vi "TagRouter.vi"(7 "Name(\"\" to use uuid)":string="UI.Dashboard") -> ()   [LabVIEW 2020, in "CSM-TagRouter.lvlib"]
doc: "------------- lvcsm -------------\n[CSMStates]\nItem 0 = \"Idle\"\nItem 1 = \"CSM Documentation\"\nItem 2 = \"VI Reference\"\nItem 3 = \"Error Handler\"\nItem 4 = \"Critical Error\"\nItem 5 = \"Target Timeout Error\"\nItem 6 = \"Target Error\"\nItem 7 = \"Async Response\"\nItem 8 = \"Response\"\nItem 9 = \"Async Message Posted\"\nItem 10 = \"Initialize Core Data\"\nItem 11 = \"Exit\"\nItem 12 = \"Data: Initialize\"\nItem 13 = \"Data: Update Indicators\"\nItem 14 = \"Data: Load Attributes\"\nItem 15 = \"Data: Save Attributes\"\nItem 16 = \"Data: Cleanup\"\nItem 17 = \"Macro: Initialize\"\nItem 18 = \"Macro: Exit\"\nItem 19 = \"API: Start Refreshing\"\nItem 20 = \"API: Stop Refreshing\"\nItem 21 = \"Action: Insert TestStandOI\"\nItem 22 = \"Action: Relocate Boolean Switchs\"\nItem 23 = \"Action: 修改bool状态\"\nItem 24 = \"Action: Sync Bool Value with DB\"\nItem 25 = \"Action: 更新当前测试名称\"\nItem 26 = \"Action: Refresh Waveform\"\nItem 27 = \"Action: Refresh Check\"\nItem 28 = \"Action: Resize Array\"\n\n[CSMStatus]\nItem 0 = \"Error Occurred@Error Handler\"\nItem 1 = \"电磁阀状态修改@Action: 修改bool状态\""
uses:
  CSM-TagRouter.lvlib
  ee6b4457-3910-401d-b6a0-627ba86d4b6e.vi
  9c140fab-bc64-4413-82a8-cd8ed97da630.vi
  82eb00db-d07c-457e-bb6f-b363662c3af2.vi
  cb63b056-b8cb-4b3f-bf45-ca82b840c7fe.vi
  edf08d9e-89a8-4fbb-bbaf-5d87ab7e3973.vi
  <userlib>/_NEVSTOP/Communicable State Machine(CSM)/AdvanceAPI/CSM - Revert Arguments-Safe String.vi
  <userlib>/_NEVSTOP/Communicable State Machine(CSM)/_Shared/Trim Single-line Text.vi
  <userlib>/_NEVSTOP/Communicable State Machine(CSM)/AdvanceAPI/CSM - Make String Arguments Safe.vi
  <userlib>/_NEVSTOP/Communicable State Machine(CSM)/AdvanceAPI/CSM - Break Down Multiple States String.vi
  <userlib>/_NEVSTOP/Communicable State Machine(CSM)/AdvanceAPI/CSM - Compact Multiple States.vi
  <userlib>/_NEVSTOP/TagDB/_Support/DataAccess/data-Write.vi
  <userlib>/_NEVSTOP/TagDB/_Support/Error/_[error50000]Invalid DB REF.vi
  <userlib>/_NEVSTOP/TagDB/_Support/DataAccess/TagDB Ref to DVR.vi
  <userlib>/_NEVSTOP/Communicable State Machine(CSM)/AdvanceAPI/CSM - Keywords.vi
  <userlib>/_NEVSTOP/TagDB/_Support/DataAccess/_NameCacher.vi
  <userlib>/_NEVSTOP/TagDB/_Support/DataAccess/_datatypeChecker.vi
  <vilib>/Utility/Data Type/Get Type Information.vi
  <userlib>/_NEVSTOP/TagDB/_Support/Error/_Build Error Cluster.vi
  <userlib>/_NEVSTOP/Communicable State Machine(CSM)/addons/MassData-Parameter/_support/FGV-MassData(lvlibp).vi
  <userlib>/_NEVSTOP/Communicable State Machine(CSM)/addons/API-String-Arugments-Support/_Support/Data To API String Arguments.vi
  <userlib>/_NEVSTOP/Communicable State Machine(CSM)/Communicable State Machine.lvlib
  <userlib>/_NEVSTOP/TagDB/TagDB.lvlib
  <userlib>/_NEVSTOP/Communicable State Machine(CSM)/addons/API-String-Arugments-Support/API String Arguments Support.lvlib
  <userlib>/_NEVSTOP/Communicable State Machine(CSM)/_Shared/CSM Shared.lvlib
panel:
  out "TagDB":refnum<k1>
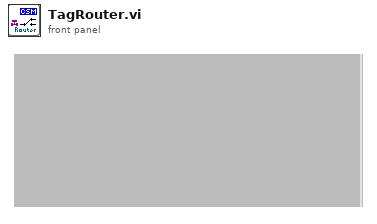
[diagram p1: front panel]
types:
  T1 = enum32{"Invalid", "Standard", "Closed", "Hidden", "Minimized", "Maximized"}
  T2 = enum32{"invalid app kind", "Development System", "Run Time System", "Student Edition", "Embedded LabVIEW", "Evaluation", "Custom"}
  T3 = typedef "Communicable State Machine.lvlib/_CSM_Response Source Message.ctl" = cluster{"‘State":string, "’Arguments":string, "’Error":errorcluster}
  T4 = cluster{"Current VI Reference":refnum<vi>, "Close Panel on Exit?":bool}
  T5 = cluster{"Core":cluster{"Current VI Reference":refnum<vi>, "Close Panel on Exit?":bool}, "Tags":string[], "Size":cluster{"Cols":i16, "Rows":i16}}
  T6 = cluster{"NI_DeviceNumber":string, "NI_ChannelName":string, "NI_LineNames":string, "NI_UnitDescription":string, "NI_ExpXDimension":string}
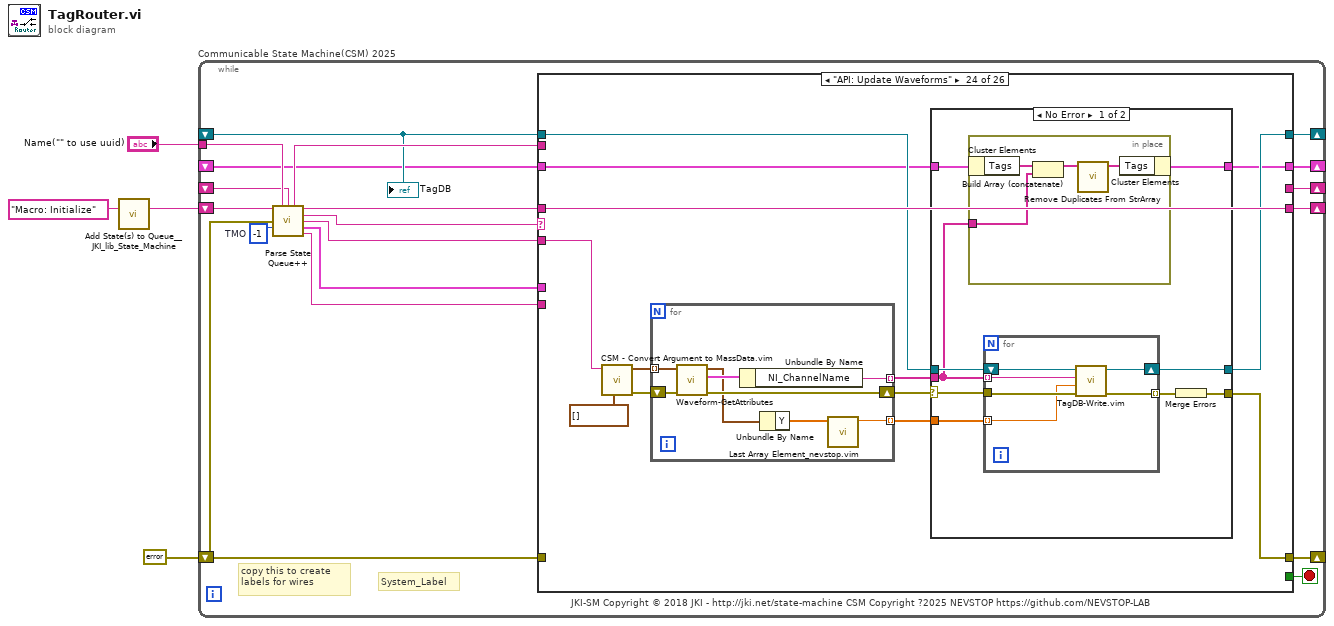
[diagram p0: block diagram]
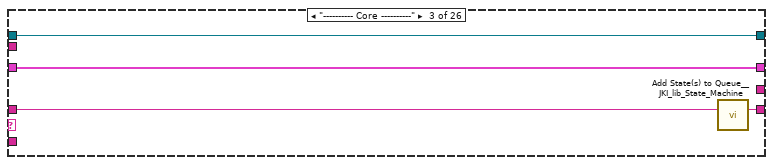
[diagram p4: hidden frame]
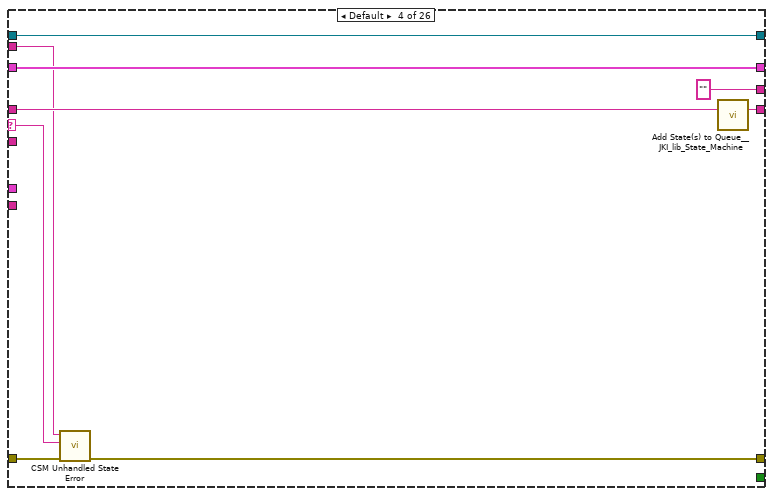
[diagram p5: hidden frame]
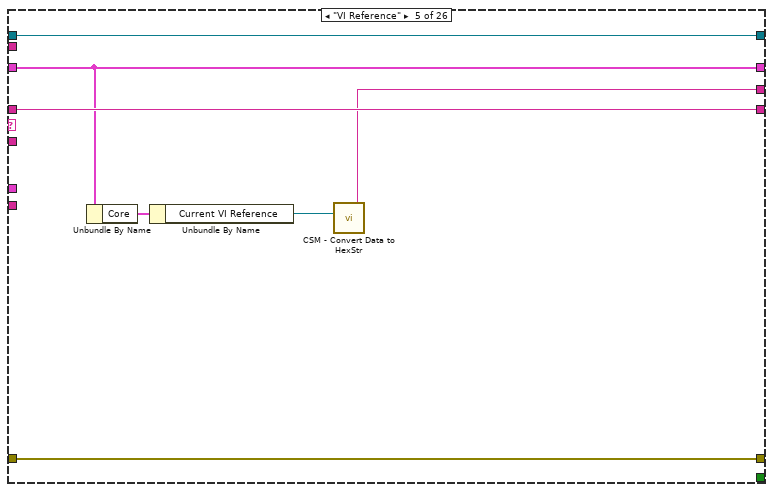
[diagram p6: hidden frame]
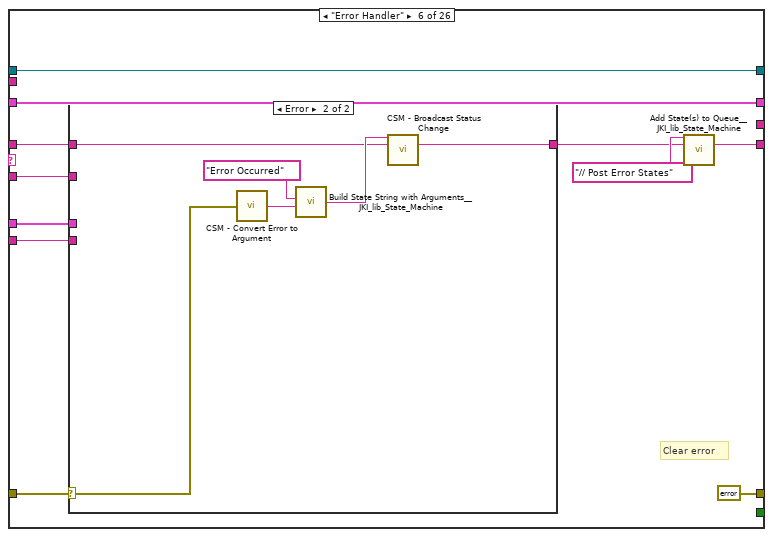
[diagram p7: hidden frame]
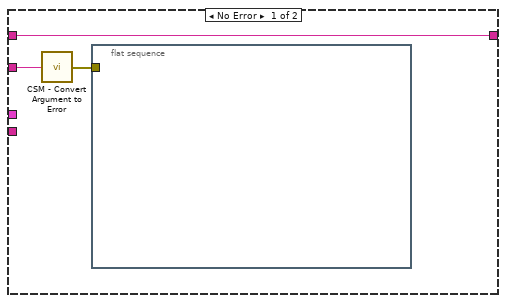
[diagram p8: hidden frame]
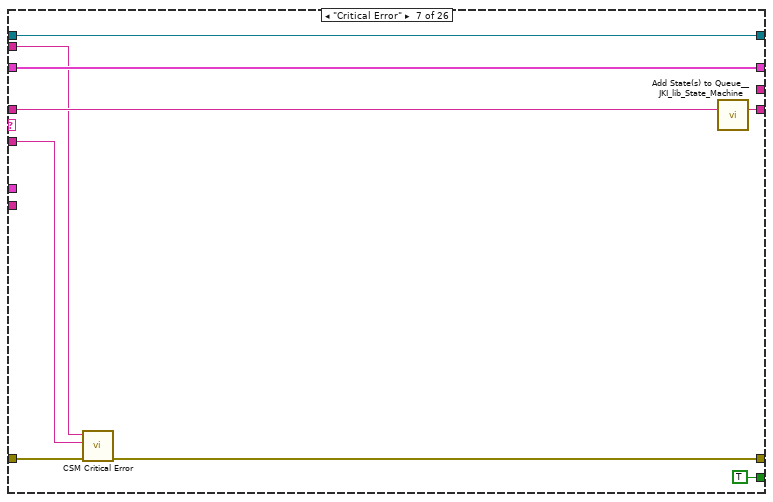
[diagram p9: hidden frame]
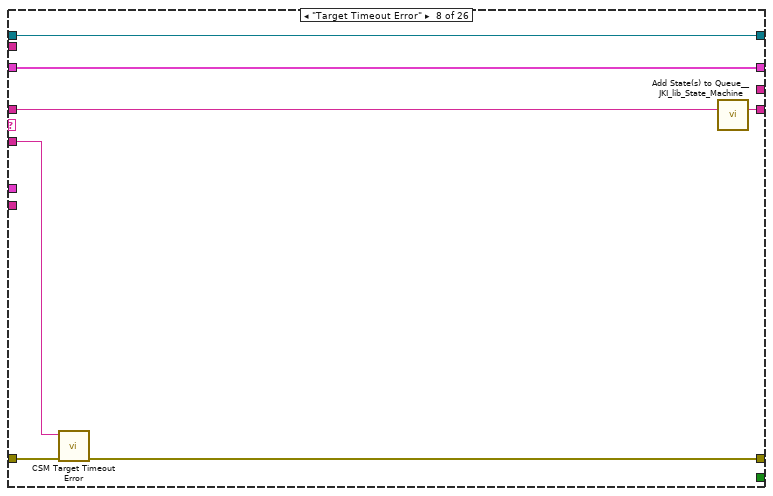
[diagram p10: hidden frame]
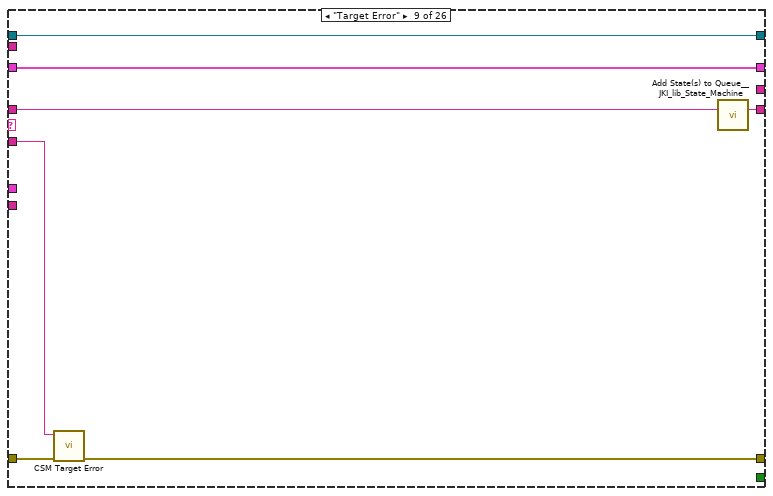
[diagram p11: hidden frame]
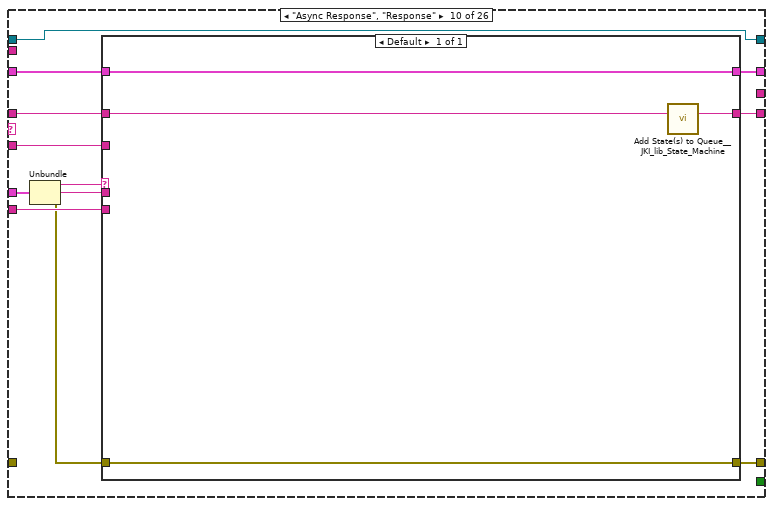
[diagram p12: hidden frame]
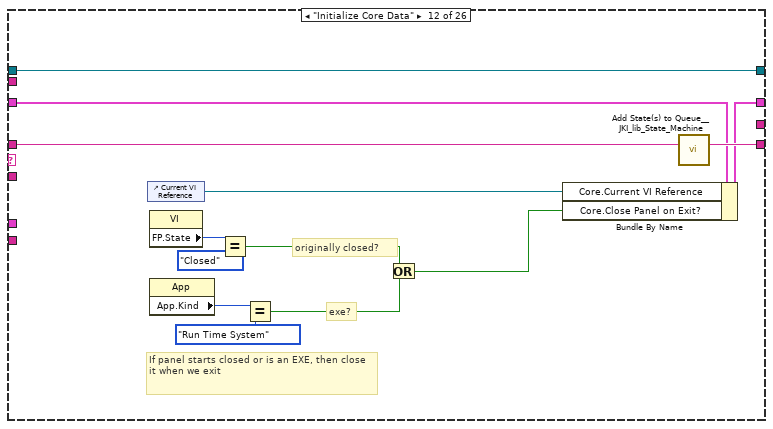
[diagram p14: hidden frame]
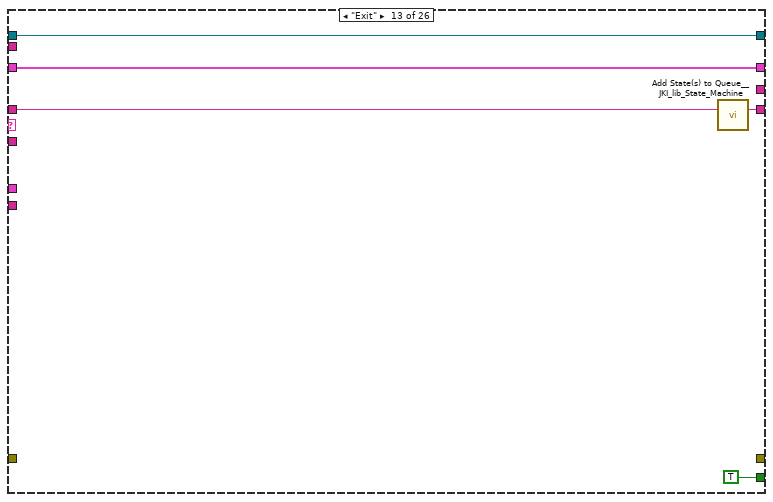
[diagram p15: hidden frame]
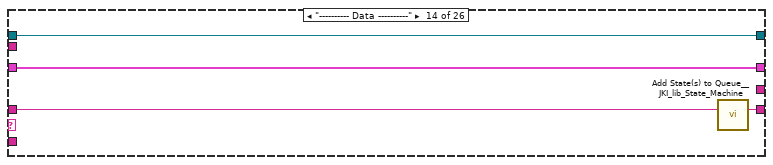
[diagram p16: hidden frame]
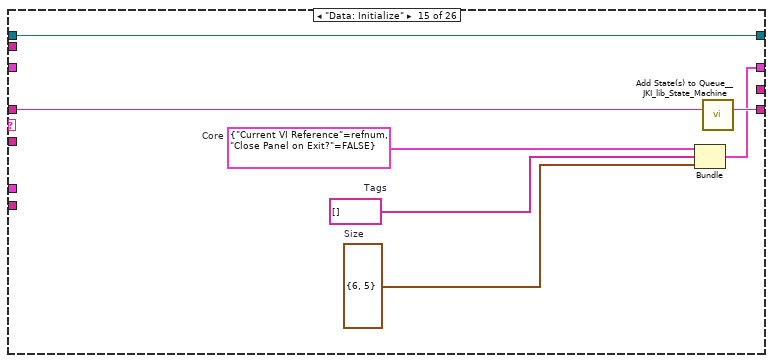
[diagram p17: hidden frame]
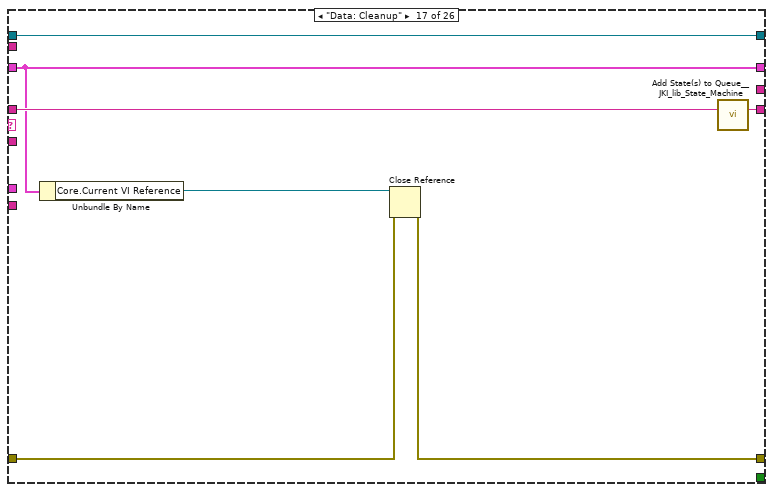
[diagram p19: hidden frame]
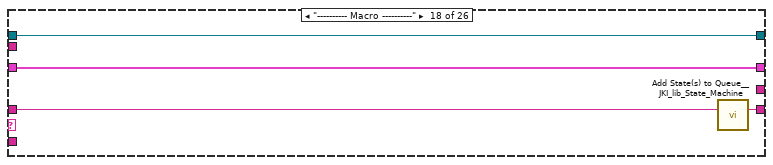
[diagram p20: hidden frame]
diagram:
  n1 = call <vilib>:"Add State(s) to Queue__JKI_lib_State_Machine.vi"("State(s) in (\"\")"="Macro: Initialize" ("Init State(\"Macro: Initialize\")")) -> ("States Out"=w4:string)  [unwired: 14 in]
  n2 = while "Communicable State Machine(CSM) 2025" {
    shift-right: [w18] -> _
    shift-left: _ -> [w5]
    shift-right: [w21] -> _
    shift-left: errorcluster {"status"=FALSE, "code"=0, "source"=""} ("error out") -> [w8]
    shift-right: [w20] -> _
    shift-left: w4 -> [w22]
    tunnel: "Name(\"\" to use uuid)" -> [w15]
    shift-right: [w16] -> _
    shift-left: _ -> [w10]
    shift-right: [w7] -> _
    shift-left: _ -> [w6]
    stop <- w19 stop-if-true
    w17 = -1  # TMO
    # "JKI-SM Copyright © 2018 JKI - http://jki.net/state-machine CSM Copyright ?2025 NEVSTOP https://github.com/NEVSTOP-LAB"
    # "copy this to create labels for wires"
    # "System_Label"
    n3 = call <userlib>:"Parse State Queue++.vi"("State Queue"=w22, "Name (\"\" to Use UUID)"=w15, "Response Arguments"=w10, "Previous Error"=w8, "Dequeue (1 ms)"=w17) -> ("Name Used"=w9:string, "Remaining States"=w23:string, "Current State"=w11:string, "Arguments"=w12:string, "Additional Information"=w13:T3, "Source CSM"=w14:string)  [unwired: 5 in]
    n4 = case shown="\"API: Update Waveforms\"" w11 {
      selector: w11 -> [_ _ _ w38 _ _ _ _ _ _ _ _ _ _ _ _ _ _ _ _ _ _ _ _ _ _]
      tunnel: w23 -> [w25 w29 w33 w42 w48 w54 w78 w85 w92 w103 w111 w124 w129 w133 w140 w143 w150 w154 w159 w166 w169 w174 w188 w233 w269 w273]
      tunnel: w12 -> [_ _ _ _ _ w53 w74 w82 w89 w97 _ _ _ _ _ _ _ _ _ _ _ w171 w186 w229 _ _]
      tunnel: w5 -> [w26 w28 w31 w40 w47 w59 w76 w83 w90 w101 w110 w118 w127 w131 _ w142 w145 w152 w157 w164 w168 w173 w187 w223 w267 w271]
      tunnel: [_ _ _ w35 w49 errorcluster {"status"=FALSE, "code"=0, "source"=""} ("error out") w71 w80 w87 w104 _ _ _ _ _ _ w146 _ _ _ _ w172 w178 w225 w264 _] -> w21
      tunnel: w8 -> [_ _ _ w36 w49 w57 w72 w81 w88 _ _ _ _ _ _ _ w147 _ _ _ _ _ _ _ _ _]
      tunnel: [w25 w29 w32 w41 w48 w55 w77 w84 w91 w102 w111 w123 w128 w132 w139 w143 w149 w153 w158 w165 w169 w174 w188 w233 w269 w272] -> w20
      tunnel: [_ _ _ _ _ _ TRUE _ _ _ _ _ TRUE _ _ _ _ _ _ _ _ _ _ _ _ _] -> w19
      tunnel: [w26 w28 w31 w40 w47 w59 w76 w83 w90 w100 w110 w122 w127 w131 w138 w142 w145 w152 w157 w164 w168 w173 w176 w222 w267 w271] -> w18
      tunnel: w14 -> [_ _ _ _ _ w52 _ _ _ w98 _ _ _ _ _ _ _ _ _ _ _ _ _ _ _ _]
      tunnel: w13 -> [_ _ _ _ _ w51 _ _ _ w99 _ _ _ _ _ _ _ _ _ _ _ _ _ _ _ _]
      tunnel: [_ _ _ "" w44 _ _ _ _ _ _ _ _ _ _ _ _ _ _ _ _ _ _ _ w265 _] -> w16
      tunnel: w9 -> [_ _ _ w37 _ _ w73 _ _ _ _ _ _ _ _ _ _ _ _ _ _ _ _ _ _ _]
      tunnel: [w24 w27 w30 w34 w43 w50 w70 w79 w86 w93 w109 w112 w125 w130 w135 w141 w144 w151 w155 w160 w167 w170 w181 w226 w268 w270] -> w7
      tunnel: w6 -> [w24 w27 w30 w34 w43 w50 w70 w79 w86 w93 w109 w112 w125 w130 w135 w141 w144 w151 w155 w160 w167 _ w182 w227 w268 w270]
      frame "", "Idle" {
      }
      frame "CSM Documentation" {
      }
      frame "---------- Core ----------" {
        n5 = call <vilib>:"Add State(s) to Queue__JKI_lib_State_Machine.vi"("State(s) in (\"\")"=w33) -> ("States Out"=w32:string)  [unwired: 14 in]
      }
      frame Default {
        n6 = call <userlib>:"CSM Unhandled State Error.vi"("error in (no error)"=w36, "Undefined State"=w38, "CSM Name"=w37) -> ("error out"=w35:errorcluster)  [unwired: 8 in]
        n7 = call <vilib>:"Add State(s) to Queue__JKI_lib_State_Machine.vi"("State(s) in (\"\")"=w42) -> ("States Out"=w41:string)  [unwired: 14 in]
      }
      frame "VI Reference" {
        n8 = Unbundle By Name(w47) -> ("Core"=w46:T4)
        n9 = Unbundle By Name(w46) -> ("Current VI Reference"=w45:refnum<vi>)
        n10 = call <userlib>:"CSM - Convert Data to HexStr.vi"("Variant"=w45) -> ("HEX String (0-9,A-F)"=w44:string)  [unwired: 8 in]
      }
      frame "Error Handler" {
        # "Clear error"
        n11 = case shown="Error" w57 {
          selector: w57 -> [_ w64]
          tunnel: [w63 w66] -> w56
          tunnel: w54 -> [w63 w65]
          tunnel: w53 -> [w62 _]
          tunnel: w52 -> [_ _]
          tunnel: w51 -> [_ _]
          frame No Error {
            n12 = call <userlib>:"CSM - Convert Argument to Error.vi"("Argument"=w62) -> ("Error"=w61:errorcluster)  [unwired: 4 in]
            n13 = flat-sequence {
              tunnel: w61 -> [_]
              frame #0 {
              }
            }
          }
          frame Error {
            n14 = call <userlib>:"CSM - Convert Error to Argument.vi"("Error"=w64) -> ("Argument"=w68:string)  [unwired: 4 in]
            n15 = call <vilib>:"Build State String with Arguments__JKI_lib_State_Machine.vi"("Arguments (\"\")"=w68, "State"="Error Occurred" ("Status with Arguments")) -> ("State with Arguments"=w67:string)  [unwired: 4 in]
            n16 = call <userlib>:"CSM - Broadcast Status Change.vi"("Status With Arguments"=w67, "State Queue"=w65) -> ("Remaining States"=w66:string)  [unwired: 13 in]
          }
        }
        n17 = call <vilib>:"Add State(s) to Queue__JKI_lib_State_Machine.vi"("State(s) in Front (\"\")"="// Post Error States", "State(s) in (\"\")"=w56) -> ("States Out"=w55:string)  [unwired: 13 in]
      }
      frame "Critical Error" {
        n18 = call <userlib>:"CSM Critical Error.vi"("error in (no error)"=w72, "Arugments (As Reason)"=w74, "CSM Name"=w73) -> ("error out"=w71:errorcluster)  [unwired: 8 in]
        n19 = call <vilib>:"Add State(s) to Queue__JKI_lib_State_Machine.vi"("State(s) in (\"\")"=w78) -> ("States Out"=w77:string)  [unwired: 14 in]
      }
      frame "Target Timeout Error" {
        n20 = call <userlib>:"CSM Target Timeout Error.vi"("error in (no error)"=w81, "Arguments (As CSM Name)"=w82) -> ("error out"=w80:errorcluster)  [unwired: 9 in]
        n21 = call <vilib>:"Add State(s) to Queue__JKI_lib_State_Machine.vi"("State(s) in (\"\")"=w85) -> ("States Out"=w84:string)  [unwired: 14 in]
      }
      frame "Target Error" {
        n22 = call <userlib>:"CSM Target Error.vi"("error in (no error)"=w88, "Arguments (As CSM Name)"=w89) -> ("error out"=w87:errorcluster)  [unwired: 9 in]
        n23 = call <vilib>:"Add State(s) to Queue__JKI_lib_State_Machine.vi"("State(s) in (\"\")"=w92) -> ("States Out"=w91:string)  [unwired: 14 in]
      }
      frame "Async Response", "Response" {
        n24 = Unbundle(w99) -> ("‘State"=w96:string, "’Arguments"=w95:string, "’Error"=w94:errorcluster)
        n25 = case shown="Default" w96 {
          tunnel: [w105] -> w102
          tunnel: w103 -> [w106]
          tunnel: [w108] -> w100
          tunnel: w101 -> [w108]
          tunnel: [w107] -> w104
          tunnel: w94 -> [w107]
          tunnel: w98 -> [_]
          tunnel: w97 -> [_]
          tunnel: w95 -> [_]
          frame Default {
            n26 = call <vilib>:"Add State(s) to Queue__JKI_lib_State_Machine.vi"("State(s) in (\"\")"=w106) -> ("States Out"=w105:string)  [unwired: 14 in]
          }
        }
      }
      frame "Async Message Posted" {
      }
      frame "Initialize Core Data" {
        # "originally closed?"
        # "exe?"
        # "If panel starts closed or is an EXE, then close it when we exit"
        n27 = control-ref of="Current VI Reference"() -> (w116:refnum<vi>)
        n28 = property class="VI"() -> ("FP.State"=w115:T1)  [unwired: 2 in, 2 out]
        n29 = property class="App"() -> ("App.Kind"=w121:T2)  [unwired: 2 in, 2 out]
        n30 = Equal?(x=w115, y=T1."Closed" ("Front Panel Window:State")) -> (x = y?=w113:bool)
        n31 = Equal?(x=w121, y=T2."Run Time System" ("Application:Kind")) -> (x = y?=w119:bool)
        n32 = Or(x=w113, y=w119) -> (x .or. y?=w117:bool)
        n33 = Bundle By Name(cluster=w118, "Core.Current VI Reference"=w116, "Core.Close Panel on Exit?"=w117) -> (w122:T5)
        n34 = call <vilib>:"Add State(s) to Queue__JKI_lib_State_Machine.vi"("State(s) in (\"\")"=w124) -> ("States Out"=w123:string)  [unwired: 14 in]
      }
      frame "Exit" {
        n35 = call <vilib>:"Add State(s) to Queue__JKI_lib_State_Machine.vi"("State(s) in (\"\")"=w129) -> ("States Out"=w128:string)  [unwired: 14 in]
      }
      frame "---------- Data ----------" {
        n36 = call <vilib>:"Add State(s) to Queue__JKI_lib_State_Machine.vi"("State(s) in (\"\")"=w133) -> ("States Out"=w132:string)  [unwired: 14 in]
      }
      frame "Data: Initialize" {
        w134 = cluster{"Cols":i16, "Rows":i16} {"Cols"=6, "Rows"=5}  # Size
        w136 = string[] []  # Tags
        w137 = T4 {"Current VI Reference"=refnum, "Close Panel on Exit?"=FALSE}  # Core
        n37 = Bundle("Core"=w137, "Tags"=w136, "Size"=w134) -> (w138:T5)  [unwired: 1 in]
        n38 = call <vilib>:"Add State(s) to Queue__JKI_lib_State_Machine.vi"("State(s) in (\"\")"=w140) -> ("States Out"=w139:string)  [unwired: 14 in]
      }
      frame "Data: Update Indicators" {
      }
      frame "Data: Cleanup" {
        n39 = Unbundle By Name(w145) -> ("Core.Current VI Reference"=w148:refnum<vi>)
        n40 = Close Reference(reference=w148, error in (no error)=w147) -> (error out=w146:errorcluster)
        n41 = call <vilib>:"Add State(s) to Queue__JKI_lib_State_Machine.vi"("State(s) in (\"\")"=w150) -> ("States Out"=w149:string)  [unwired: 14 in]
      }
      frame "---------- Macro ----------" {
        n42 = call <vilib>:"Add State(s) to Queue__JKI_lib_State_Machine.vi"("State(s) in (\"\")"=w154) -> ("States Out"=w153:string)  [unwired: 14 in]
      }
      frame "Macro: Initialize" {
        n43 = call <vilib>:"Add State(s) to Queue__JKI_lib_State_Machine.vi"("State(s) in Front (\"\")"="Data: Initialize\nInitialize Core Data\nData: Update Indicators", "State(s) in (\"\")"=w159) -> ("States Out"=w158:string)  [unwired: 13 in]
      }
      frame "Macro: Exit" {
        n44 = call <vilib>:"Add State(s) to Queue__JKI_lib_State_Machine.vi"("State(s) in Front (\"\")"="//Exit Sub-Modules ", "State(s) at Back (\"\")"="Data: Cleanup\nExit") -> ("States Out"=w162:string)  [unwired: 13 in]
        n45 = call <vilib>:"Add State(s) to Queue__JKI_lib_State_Machine.vi"("State(s) in Front (\"\")"=w162, "State(s) in (\"\")"=w166) -> ("States Out"=w165:string)  [unwired: 13 in]
      }
      frame "---------- API ----------" {
      }
      frame "API: Set TagDB" {
        n46 = call <userlib>:"TagDB-Obtain.vi"("name (unnamed)"=w171) -> ("error out"=w172:errorcluster, "TagDB"=w170:refnum<k1>)  [unwired: 4 in, 1 out]
      }
      frame "API: Update Value", "API: Update Values" {
        n47 = call <userlib>:"String to 1D Array_csm.vi"("delimiter (Tab)"=";", "string"=w186) -> ("Array of Strings"=w184:string[])  [unwired: 9 in]
        n48 = for {
          tunnel: w184 -> [w220] mode=indexing
          tunnel: [w218] -> w175 mode=indexing
          tunnel: [w217] -> w180 mode=indexing
          tunnel: [w215] -> w183 mode=indexing
          n49 = Match Pattern(string=w220, regular expression=":" ("delimiter (Tab)")) -> (before substring=w218:string, after substring=w217:string, offset past match=w216:i32)  [unwired: 1 in, 1 out]
          n50 = Greater Or Equal To 0?(x=w216) -> (x >= 0?=w215:bool)
        }
        n51 = And Array Elements(Boolean array=w183) -> (logical AND=w177:bool)
        n52 = case shown="False" w177 {
          tunnel: [w214 _] -> w179
          frame False {
            n53 = call <userlib>:"Build Error Cluster.vi"("String to Prepend to Source (\"\")"="Not valid format" ("String to Prepend to Source (\"\")"), "Code"=-1) -> ("error out"=w214:errorcluster)
          }
          frame True {
          }
        }
        n54 = case shown="No Error" w179 {
          selector: w179 -> [w192 w209]
          tunnel: w187 -> [w197 w211]
          tunnel: w182 -> [w196 w210]
          tunnel: [w195 w210] -> w181
          tunnel: w180 -> [w194 _]
          tunnel: [w191 w209] -> w178
          tunnel: [w190 w211] -> w176
          tunnel: w175 -> [w189 _]
          frame No Error {
            n55 = in-place {
              in-place-border: w189 -> [w199]
              n56 = in-place-cluster #1(w197) -> ("Tags"=w201:string[])
              n57 = Build Array (concatenate)(w201, w199) -> (w200:string[])
              n58 = call <userlib>:"Remove Duplicates From StrArray.vi"("StrArray In"=w200) -> ("StrArray"=w198:string[])  [unwired: 9 in, 1 out]
              n59 = in-place-cluster #1("Tags"=w198) -> (w190:T5)
            }
            n60 = for {
              tunnel: w189 -> [w206] mode=indexing
              shift-right: [w207] -> w195
              shift-left: w196 -> [w208]
              tunnel: w194 -> [w205] mode=indexing
              tunnel: [w204] -> w193 mode=indexing
              tunnel: w192 -> [w203]
              n61 = call <userlib>:"String To Float_csm.vi"("String"=w205) -> ("Float"=w202:dbl)  [unwired: 3 in, 1 out]
              n62 = call "TagDB-Write.vim"("error in (no error)"=w203, "Value"=w202, "tag"=w206, "TagDB"=w208) -> ("error out"=w204:errorcluster, "TagDB(dup)"=w207:refnum<k1>)  [unwired: 5 in, 1 out]
            }
            n63 = Merge Errors(w193) -> (w191:errorcluster)
          }
          frame Error {
          }
        }
      }
      frame "API: Update Waveforms" {
        n64 = call "CSM - Convert Argument to MassData.vim"("Type"=waveform(dbl)[] [] ("Graph"), "MassData Argument"=w229) -> ("error out"=w230:errorcluster, "Data"=w231:waveform(dbl)[])  [unwired: 6 in]
        n65 = for {
          tunnel: w231 -> [w263] mode=indexing
          shift-right: [w261] -> w228
          shift-left: w230 -> [w262]
          tunnel: [w258] -> w221 mode=indexing
          tunnel: [w256] -> w224 mode=indexing
          n66 = call "Waveform-GetAttributes.vi"("error in (no error)"=w262, "signal in"=w263) -> ("error out"=w261:errorcluster, "WaveformInfo"=w260:T6, "signal out"=w259:waveform(dbl))  [unwired: 7 in]
          n67 = Unbundle By Name(w260) -> ("NI_ChannelName"=w258:string)
          n68 = Unbundle By Name(w259) -> ("Y"=w257:dbl[])
          n69 = call "Last Array Element_nevstop.vim"("Array"=w257) -> ("Last Element"=w256:dbl)  [unwired: 10 in]
        }
        n70 = case shown="No Error" w228 {
          selector: w228 -> [w241 w255]
          tunnel: w227 -> [w240 w254]
          tunnel: [w239 w254] -> w226
          tunnel: [w238 w255] -> w225
          tunnel: w224 -> [w237 _]
          tunnel: w223 -> [w236 w253]
          tunnel: [w235 w253] -> w222
          tunnel: w221 -> [w234 _]
          frame No Error {
            n71 = in-place {
              in-place-border: w234 -> [w244]
              n72 = in-place-cluster #2(w236) -> ("Tags"=w246:string[])
              n73 = Build Array (concatenate)(w246, w244) -> (w245:string[])
              n74 = call <userlib>:"Remove Duplicates From StrArray.vi"("StrArray In"=w245) -> ("StrArray"=w243:string[])  [unwired: 9 in, 1 out]
              n75 = in-place-cluster #2("Tags"=w243) -> (w235:T5)
            }
            n76 = for {
              tunnel: w234 -> [w250] mode=indexing
              shift-right: [w251] -> w239
              shift-left: w240 -> [w252]
              tunnel: [w249] -> w242 mode=indexing
              tunnel: w241 -> [w248]
              tunnel: w237 -> [w247] mode=indexing
              n77 = call "TagDB-Write.vim"("error in (no error)"=w248, "Value"=w247, "tag"=w250, "TagDB"=w252) -> ("error out"=w249:errorcluster, "TagDB(dup)"=w251:refnum<k1>)  [unwired: 5 in, 1 out]
            }
            n78 = Merge Errors(w242) -> (w238:errorcluster)
          }
          frame Error {
          }
        }
      }
      frame "API: Tags" {
        n79 = Unbundle By Name(w267) -> ("Tags"=w266:string[])
        n80 = call "Convert Data To API String Arguments.vim"("Data"=w266) -> ("error out"=w264:errorcluster, "API String"=w265:string)  [unwired: 7 in]
      }
      frame "---------- Action ----------" {
        n81 = call <vilib>:"Add State(s) to Queue__JKI_lib_State_Machine.vi"("State(s) in (\"\")"=w273) -> ("States Out"=w272:string)  [unwired: 14 in]
      }
    }
    "TagDB" <- w6
  }
